vi "CSDB_Config.database.vi"(0 "connectionRef":T1, 1 "setReference":bool, 5 "error in (no error)":errorcluster) -> (14 "connectionRef out":T1, 19 "error out":errorcluster)   [LabVIEW 2014, in "CSDB_Config.lvlib"]
doc: "Sets/Gets the connection reference to a database"
uses:
  CSDB_Config.lvlib
  <vilib>/addons/database/Connection.llb/Conn ObjectReference.ctl
  <vilib>/addons/database/NI_Database_API.lvlib
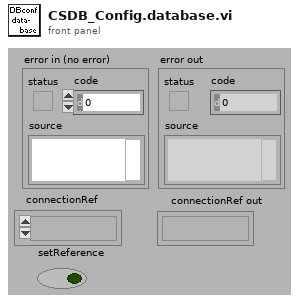
[diagram p1: front panel]
types:
  T1 = typedef "NI_Database_API.lvlib/Conn ObjectReference.ctl" = refnum<k1>
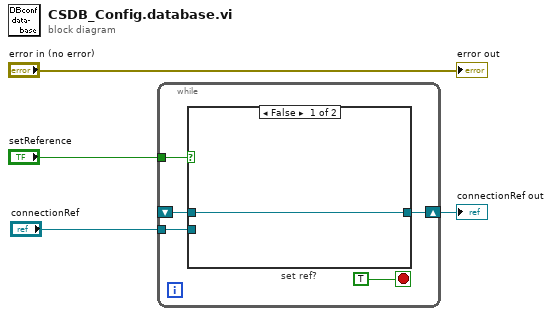
[diagram p0: block diagram]
diagram:
  n1 = while {
    tunnel: "setReference" -> [w8]
    shift-right: [w6] -> w2
    shift-left: _ -> [w5]
    tunnel: "connectionRef" -> [w7]
    stop <- TRUE stop-if-true
    n2 = case "set ref?" shown="False" w8 {
      tunnel: [w10 w11] -> w6
      tunnel: w7 -> [_ w11]
      tunnel: w5 -> [w10 _]
      frame False {
      }
      frame True {
      }
    }
  }
  "connectionRef out" <- w2
  "error out" <- "error in (no error)"
